vi "draw.vi"(0 "reference":refnum<class "MultiLineString.lvclass">, 1 "graphics":refnum<class "Graphics.lvclass">, 2 "bounds":T1 {"height" format="%.2f"; "width" format="%.2f"; "y" format="%.2f"; "x" format="%.2f"}, 5 "error in (no error)":errorcluster) -> (14 "reference out":refnum<class "MultiLineString.lvclass">, 19 "error out":errorcluster)   [LabVIEW 2020, in "MultiLineString.lvclass"]
doc: "public void draw(Graphics2D g2, Rectangle2D r)"
uses:
  <resource>/Framework/Providers/Open_GDS/UML/MultiLineString_class/MultiLineString.lvclass
  <resource>/Framework/Providers/Open_GDS/UML/Graphics_class/Graphics.lvclass
  <resource>/Framework/Providers/Open_GDS/UML/General/Rectangle/Rectangle Rectangle2D.ctl
  <resource>/Framework/Providers/Open_GDS/UML/General/Point/Point Point2D.ctl
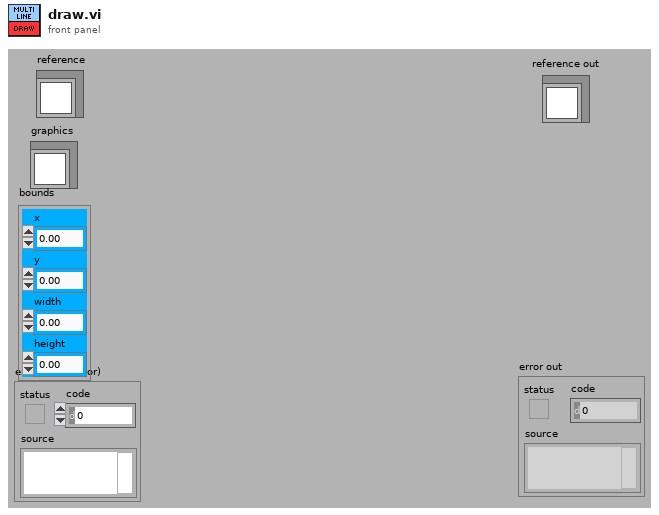
[diagram p1: front panel]
types:
  T1 = typedef "Rectangle Rectangle2D.ctl" = cluster{"x":dbl, "y":dbl, "width":dbl, "height":dbl}
  T2 = typedef "Point Point2D.ctl" = cluster{"x":dbl, "y":dbl}
  T3 = typedef "MultiLineString.lvclass/ObjectAttributes.ctl" = cluster{"GAP":i32, "text":string, "justification":T4, "size":T5, "underlined":bool}
  T4 = typedef "MultiLineString.lvclass/JustificationType.ctl" = enum16{"LEFT", "CENTER", "RIGHT"}
  T5 = typedef "MultiLineString.lvclass/SizeType.ctl" = enum16{"LARGE", "NORMAL", "SMALL"}
  T6 = typedef "Graphics.lvclass/LvFontType.ctl" = enum16{"User-specified Font", "Application Font", "System Font", "Dialog Font"}
  T7 = typedef "Graphics.lvclass/FontType.ctl" = cluster{"Font Name:":string, "Size":i16, "Strikeout?":bool, "Italic?":bool, "Underline?":bool, "Outline?":bool, "Shadow?":bool, "Bold?":bool}
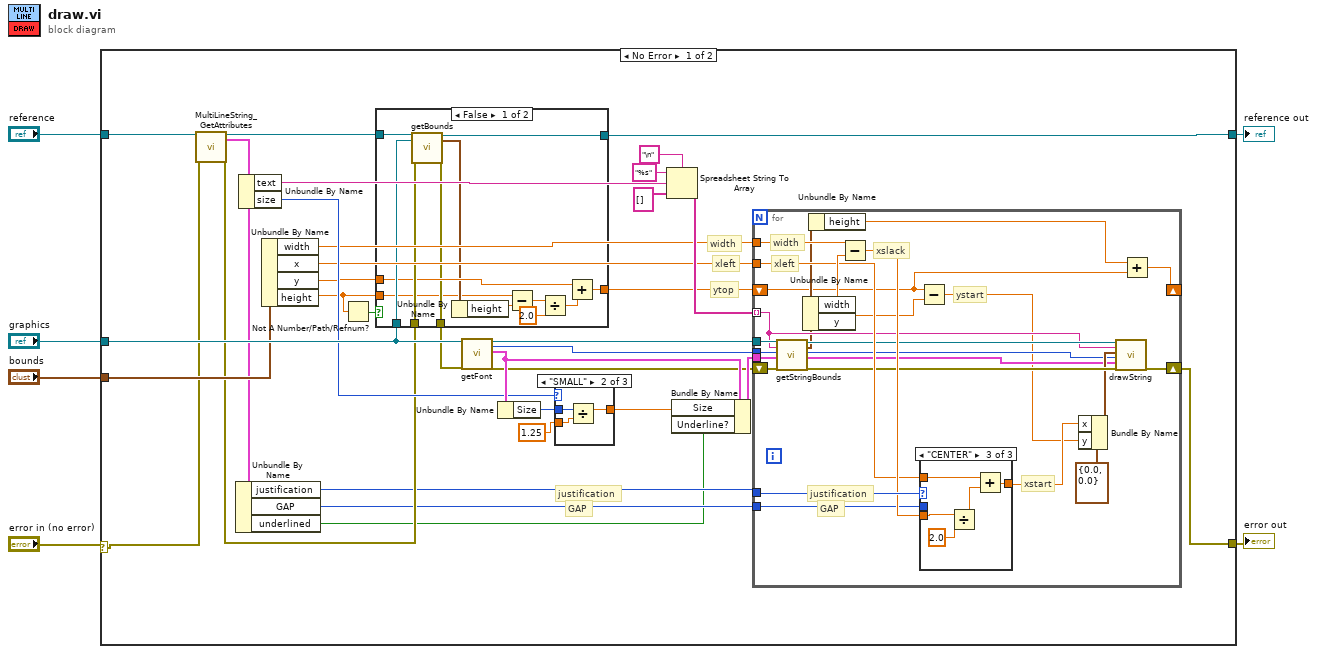
[diagram p0: block diagram]
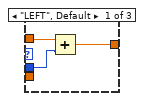
[diagram p3: hidden frame]
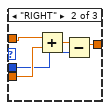
[diagram p4: hidden frame]
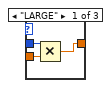
[diagram p5: hidden frame]
diagram:
  n1 = case shown="No Error" "error in (no error)" {
    selector: "error in (no error)" -> [w34 w99]
    tunnel: "reference" -> [w39 w100]
    tunnel: [w38 w99] -> w5
    tunnel: [w37 w100] -> w4
    tunnel: "graphics" -> [w36 _]
    tunnel: "bounds" -> [w35 _]
    frame No Error {
      # "GAP"
      # "justification"
      # "width"
      # "xleft"
      # "ytop"
      n2 = call <resource>:"MultiLineString_GetAttributes.vi"("reference in"=w39, "error in (no error)"=w34) -> ("reference out"=w33:refnum<class "MultiLineString.lvclass">, "Data"=w7:T3, "error out"=w18:errorcluster)  [unwired: 1 in, 14 out]
      n3 = Unbundle By Name(w7) -> ("justification"=w14:T4, "GAP"=w13:i32, "underlined"=w12:bool)
      n4 = Unbundle By Name(w7) -> ("text"=w20:string, "size"=w19:T5)
      n5 = Unbundle By Name(w35) -> ("width"=w15:dbl, "x"=w16:dbl, "y"=w17:dbl, "height"=w8:dbl)
      n6 = Not A Number/Path/Refnum?(number/path/refnum=w8) -> (NaN/Path/Refnum?=w9:bool)
      n7 = case shown="False" w9 {
        tunnel: [w52 w55] -> w37
        tunnel: w36 -> [w51 _]
        tunnel: w33 -> [w50 w55]
        tunnel: w18 -> [w49 w54]
        tunnel: w17 -> [w48 w53]
        tunnel: [w42 w53] -> w11
        tunnel: [w41 w54] -> w10
        tunnel: w8 -> [w40 _]
        frame False {
          n8 = call-dynamic "getBounds.vi"("reference"=w50, "graphics"=w51, "error in (no error)"=w49) -> ("reference out"=w52:refnum<class "MultiLineString.lvclass">, "bounds"=w47:T1, "error out"=w41:errorcluster)  [unwired: 14 out]
          n9 = Unbundle By Name(w47) -> ("height"=w46:dbl)
          n10 = Subtract(x=w40, y=w46) -> (x-y=w45:dbl)
          n11 = Divide(x=w45, y=2.0) -> (x/y=w44:dbl)
          n12 = Add(x=w48, y=w44) -> (x+y=w42:dbl)
        }
        frame True {
        }
      }
      n13 = call <resource>:"getFont.vi"("reference"=w36, "error in (no error)"=w10) -> ("reference out"=w32:refnum<class "Graphics.lvclass">, "fontType"=w31:T6, "font"=w28:T7, "error out"=w21:errorcluster)  [unwired: 14 out]
      n14 = Unbundle By Name(w28) -> ("Size"=w30:i16)
      n15 = case shown="\"SMALL\"" w19 {
        tunnel: w30 -> [w94 w96 w98]
        tunnel: 1.25 ("y") -> [w93 w97 _]
        tunnel: [w92 w95 w98] -> w26
        frame "LARGE" {
          n16 = Multiply(x=w94, y=w93) -> (x*y=w92:dbl)
        }
        frame "SMALL" {
          n17 = Divide(x=w96, y=w97) -> (x/y=w95:dbl)
        }
        frame "NORMAL", Default {
        }
      }
      n18 = Spreadsheet String To Array(delimiter (Tab)="\n", format string="%s", spreadsheet string=w20, array type (2D Dbl)=string[] []) -> (array=w22:string[])
      n19 = Bundle By Name(cluster=w28, "Size"=w26, "Underline?"=w12) -> (w27:T7)
      n20 = for {
        tunnel: w32 -> [w78]
        tunnel: w31 -> [w63]
        tunnel: w27 -> [w62]
        tunnel: w22 -> [w64] mode=indexing
        shift-right: [w67] -> w38
        shift-left: w21 -> [w77]
        tunnel: w16 -> [w72]
        tunnel: w15 -> [w76]
        tunnel: w14 -> [w74]
        tunnel: w13 -> [w71]
        shift-right: [w59] -> _
        shift-left: w11 -> [w56]
        # "ystart"
        # "xstart"
        # "xleft"
        # "width"
        # "justification"
        # "GAP"
        # "xslack"
        n21 = call-dynamic "getStringBounds.vi"("reference"=w78, "text"=w64, "fontType"=w63, "font"=w62, "error in (no error)"=w77) -> ("reference out"=w69:refnum<class "Graphics.lvclass">, "bounds"=w58:T1, "error out"=w68:errorcluster)  [unwired: 12 out]
        n22 = Unbundle By Name(w58) -> ("width"=w75:dbl, "y"=w70:dbl)
        n23 = Unbundle By Name(w58) -> ("height"=w57:dbl)
        n24 = Subtract(x=w76, y=w75) -> (x-y=w73:dbl)
        n25 = Subtract(x=w56, y=w70) -> (x-y=w60:dbl)
        n26 = case shown="\"CENTER\"" w74 {
          tunnel: w73 -> [_ w85 w90]
          tunnel: w72 -> [w81 w86 w88]
          tunnel: w71 -> [w80 w83 _]
          tunnel: [w79 w82 w87] -> w61
          frame "LEFT", Default {
            n27 = Add(x=w81, y=w80) -> (x+y=w79:dbl)
          }
          frame "RIGHT" {
            n28 = Add(x=w86, y=w85) -> (x+y=w84:dbl)
            n29 = Subtract(x=w84, y=w83) -> (x-y=w82:dbl)
          }
          frame "CENTER" {
            n30 = Divide(x=w90, y=2.0) -> (x/y=w89:dbl)
            n31 = Add(x=w88, y=w89) -> (x+y=w87:dbl)
          }
        }
        n32 = Bundle By Name(cluster=T2 {"x"=0.0, "y"=0.0} ("textPos"), "x"=w61, "y"=w60) -> (w65:T2)
        n33 = call-dynamic "drawString.vi"("reference"=w69, "text"=w64, "textPos"=w65, "fontType"=w63, "font"=w62, "error in (no error)"=w68) -> ("error out"=w67:errorcluster)  [unwired: 1 in, 12 out]
        n34 = Add(x=w57, y=w56) -> (x+y=w59:dbl)
      }
    }
    frame Error {
    }
  }
  "reference out" <- w4
  "error out" <- w5
